vi "Boolean Crossing.vi"(1 "Initialize":bool, 2 "Direction":enum8{"Either", "False-True", "True-False"}(ring), 3 "Input":bool) -> (0 "Crossing":bool)   [LabVIEW 2019]
doc: "Detects transitions of <B> Input </B>. You can choose one of the following directions: <B> Either </B>, <B> False-True </B> or <B> True-False </B>."
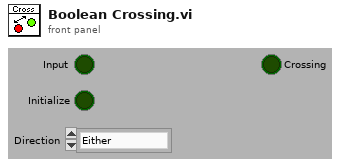
[diagram p1: front panel]
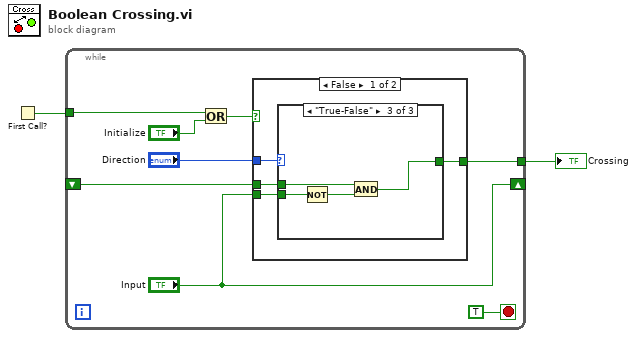
[diagram p0: block diagram]
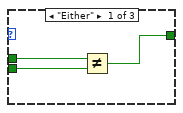
[diagram p2: hidden frame]
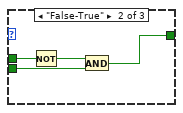
[diagram p3: hidden frame]
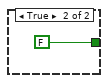
[diagram p4: hidden frame]
diagram:
  n1 = First Call?() -> (First Call?: T/F=w2:bool)
  n2 = while {
    tunnel: w2 -> [w9]
    tunnel: [w5] -> w1
    shift-right: ["Input"] -> _
    shift-left: _ -> [w4]
    stop <- TRUE stop-if-true
    n3 = Or(x=w9, y="Initialize") -> (x .or. y?=w8:bool)
    n4 = case shown="False" w8 {
      tunnel: "Direction" -> [w14 _]
      tunnel: [w13 FALSE] -> w5
      tunnel: w4 -> [w12 _]
      tunnel: "Input" -> [w11 _]
      frame False {
        n5 = case shown="\"True-False\"" w14 {
          tunnel: [w17 w21 w25] -> w13
          tunnel: w12 -> [w16 w20 w23]
          tunnel: w11 -> [w15 w19 w24]
          frame "Either" {
            n6 = Not Equal?(x=w16, y=w15) -> (x != y?=w17:bool)
          }
          frame "False-True" {
            n7 = Not(x=w20) -> (.not. x?=w18:bool)
            n8 = And(x=w18, y=w19) -> (x .and. y?=w21:bool)
          }
          frame "True-False" {
            n9 = Not(x=w24) -> (.not. x?=w22:bool)
            n10 = And(x=w23, y=w22) -> (x .and. y?=w25:bool)
          }
        }
      }
      frame True {
      }
    }
  }
  "Crossing" <- w1
